vi "x-axis.vi"(8 "error in (no error)":errorcluster, 11 "Pulse Gen Scan in":refnum<class "Pulse Gen Scan.lvclass">) -> (0 "error out":errorcluster, 1 "Label":string, 2 "Unit":string, 3 "Pulse Gen Scan out":refnum<class "Pulse Gen Scan.lvclass">)   [LabVIEW 2012, in "Pulse Gen Scan.lvclass"]
uses:
  Pulse Gen Scan.lvclass
  Scanner/Scanner.lvclass
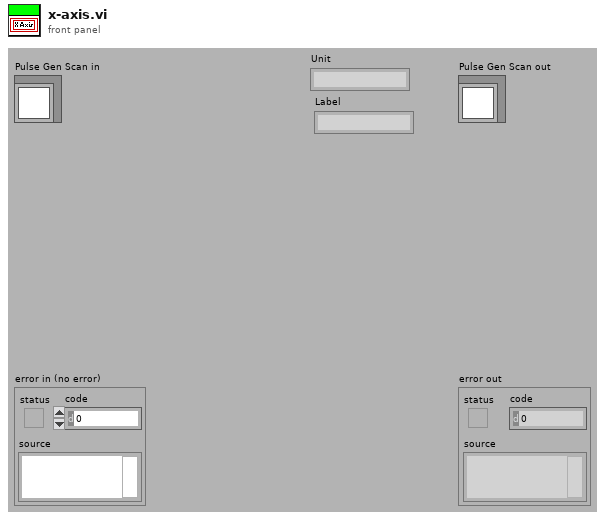
[diagram p1: front panel]
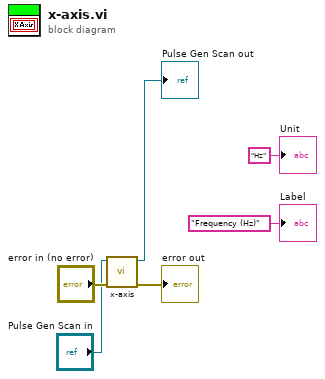
[diagram p0: block diagram]
diagram:
  n1 = call-parent "x-axis.vi"("error in (no error)"="error in (no error)", "Scanner in"="Pulse Gen Scan in") -> ("error out"=→"error out":errorcluster, "Scanner out"=→"Pulse Gen Scan out":refnum<class "Pulse Gen Scan.lvclass">)  [unwired: 6 in, 2 out]
  "Label" <- "Frequency (Hz)" ("Label")
  "Unit" <- "Hz" ("Unit")
